vi "Repack Pixels_Pixel Bus to FIFO U1x8.vi"(10 "Input Valid":bool=TRUE, 11 "Pixel Bus In":T1={"Pixel Data"=[FALSE, FALSE, FALSE, FALSE, FALSE, FALSE, FALSE, FALSE], "DV"=[FALSE, FALSE, FALSE, FALSE, FALSE, FALSE, FALSE, FALSE], "EOL"=FALSE, "EOI"=FALSE, "Data Type"=enum."U1 x 8"}) -> (2 "Output Valid":bool, 3 "output array":bool[](array[boolean]))   [LabVIEW 2020, in "NI_VDM_FPGA_Basics.lvlib"]
uses:
  <vilib>/visionFPGA/NI_VDM_FPGA_Basics.lvlib
  <vilib>/visionFPGA/Controls/IMAQ FPGA Pixel Bus u1x8.ctl
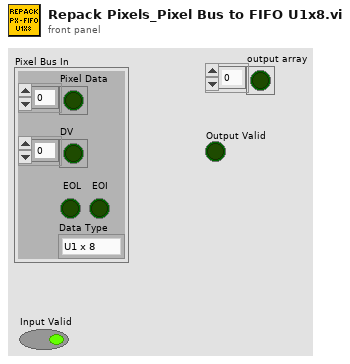
[diagram p1: front panel]
types:
  T1 = typedef "IMAQ FPGA Pixel Bus u1x8.ctl" = cluster{"Pixel Data":bool[], "DV":bool[], "EOL":bool, "EOI":bool, "Data Type":enum16{"U1 x 8"}}
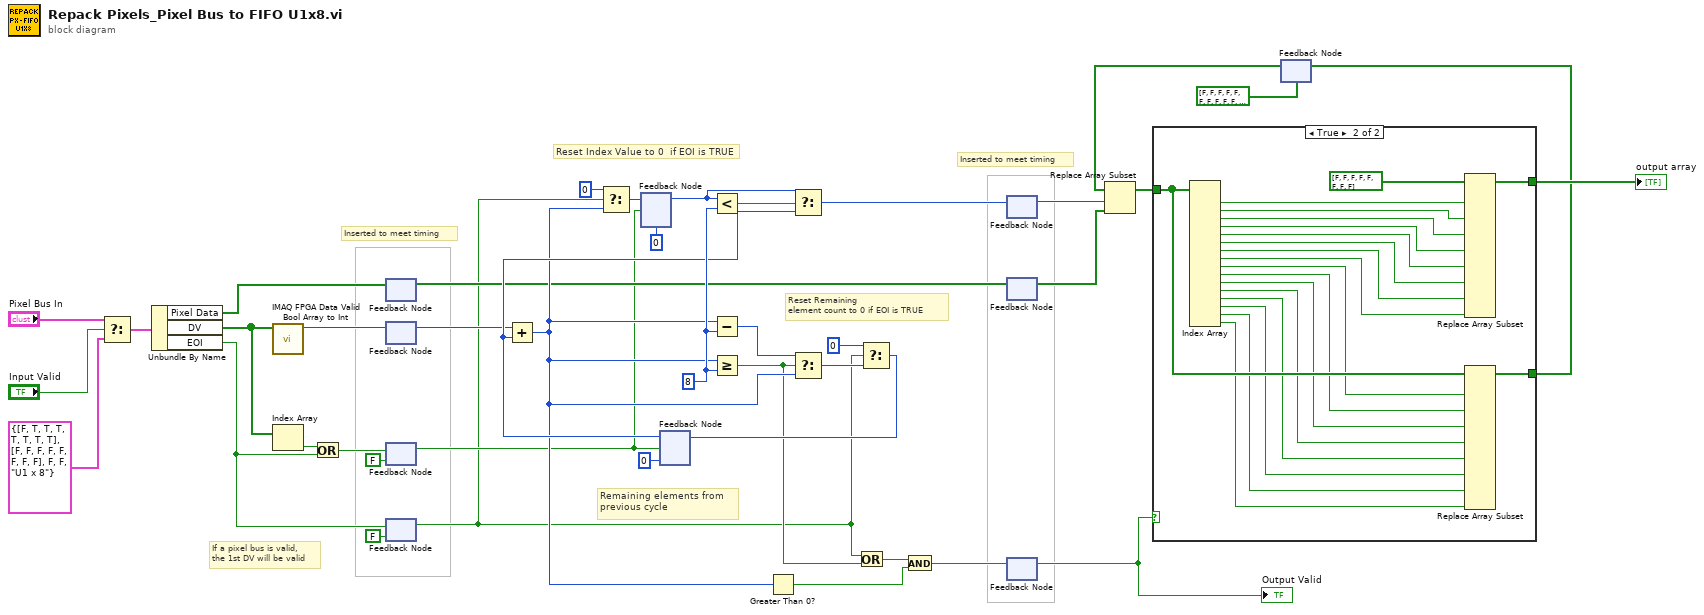
[diagram p0: block diagram]
diagram:
  w32 = u16 8 ("y")
  # "Inserted to meet timing"
  # "If a pixel bus is valid,\nthe 1st DV will be valid"
  # "Inserted to meet timing"
  # "Reset Remaining \nelement count to 0 if EOI is TRUE"
  # "Reset Index Value to 0  if EOI is TRUE"
  # "Remaining elements from \nprevious cycle"
  n1 = Select(t="Pixel Bus In", s="Input Valid", f=T1 {"Pixel Data"=[FALSE, TRUE, TRUE, TRUE, TRUE, TRUE, TRUE, TRUE], "DV"=[FALSE, FALSE, FALSE, FALSE, FALSE, FALSE, FALSE, FALSE], "EOL"=FALSE, "EOI"=FALSE, "Data Type"=enum."U1 x 8"} ("Pixel Bus In")) -> (s? t:f=w39:T1)
  n2 = Unbundle By Name(w39) -> ("Pixel Data"=w16:bool[], "DV"=w15:bool[], "EOI"=w9:bool)
  n3 = call <vilib>:"IMAQ FPGA Data Valid Bool Array to Int.vi"("DV In"=w15) -> ("Sum DV Out"=w28:u8)  [unwired: 10 in]
  n4 = Index Array(array=w15) -> (element=w17:bool)  [unwired: 1 in]
  n5 = Or(x=w17, y=w9) -> (x .or. y?=w12:bool)
  n6 = feedback-in #1(w16) -> ()
  n7 = feedback #1() -> (w14:bool[])  [unwired: 1 in]
  n8 = feedback-in #2(w28) -> ()
  n9 = feedback #2() -> (w13:u8)  [unwired: 1 in]
  n10 = feedback #3(FALSE) -> (w8:bool)
  n11 = feedback-in #3(w12) -> ()
  n12 = feedback #4(FALSE) -> (w1:bool)
  n13 = feedback-in #4(w9) -> ()
  n14 = feedback #5(u16 0 ("t")) -> (w31:u16)
  n15 = feedback #6(u16 0 ("t")) -> (w27:u16)
  n16 = Add(x=w13, y=w27) -> (x+y=w20:u16)
  n17 = Select(t=u16 0, s=w1, f=w20) -> (s? t:f=w22:u16)
  n18 = feedback-in #5(w22, w8) -> ()
  n19 = Less?(x=w31, y=w32) -> (x < y?=w29:bool)
  n20 = Subtract(x=w20, y=w32) -> (x-y=w33:u16)
  n21 = Greater Or Equal?(x=w20, y=w32) -> (x >= y?=w2:bool)
  n22 = Greater Than 0?(x=w20) -> (x > 0?=w19:bool)
  n23 = Select(t=w31, s=w29, f=w27) -> (s? t:f=w30:u16)
  n24 = Select(t=w33, s=w2, f=w20) -> (s? t:f=w25:u16)
  n25 = Or(x=w1, y=w2) -> (x .or. y?=w26:bool)
  n26 = Select(t=u16 0, s=w1, f=w25) -> (s? t:f=w23:u16)
  n27 = feedback-in #6(w23, w8) -> ()
  n28 = And(x=w26, y=w19) -> (x .and. y?=w42:bool)
  n29 = feedback-in #7(w30) -> ()
  n30 = feedback #7() -> (w6:u16)  [unwired: 1 in]
  n31 = feedback-in #8(w14) -> ()
  n32 = feedback #8() -> (w7:bool[])  [unwired: 1 in]
  n33 = feedback-in #9(w42) -> ()
  n34 = feedback #9() -> (w5:bool)  [unwired: 1 in]
  "Output Valid" <- w5
  n35 = feedback #10(bool[] [FALSE, FALSE, FALSE, FALSE, FALSE, FALSE, FALSE, FALSE, FALSE, FALSE, FALSE, FALSE, FALSE, FALSE, FALSE, FALSE] ("Pixel Data")) -> (w35:bool[])
  n36 = Replace Array Subset(array=w35, new element=w7, index=w6) -> (w34:bool[])
  n37 = case shown="True" w5 {
    tunnel: [w43 w63] -> w36
    tunnel: w34 -> [w43 w62]
    tunnel: [_ w45] -> w37
    frame False {
    }
    frame True {
      n38 = Index Array(array=w62) -> (element #1=w61:bool, element #2=w60:bool, element #3=w59:bool, element #4=w58:bool, element #5=w57:bool, element #6=w56:bool, element #7=w55:bool, element #8=w54:bool, element #9=w53:bool, element #10=w52:bool, element #11=w51:bool, element #12=w50:bool, element #13=w49:bool, element #14=w48:bool, element #15=w47:bool, element #16=w46:bool)  [unwired: 16 in]
      n39 = Replace Array Subset(array=bool[] [FALSE, FALSE, FALSE, FALSE, FALSE, FALSE, FALSE, FALSE] ("Pixel Data"), new element #1=w61, new element #2=w60, new element #3=w59, new element #4=w58, new element #5=w57, new element #6=w56, new element #7=w55, new element #8=w54) -> (w45:bool[])  [unwired: 8 in]
      n40 = Replace Array Subset(array=w62, new element #1=w53, new element #2=w52, new element #3=w51, new element #4=w50, new element #5=w49, new element #6=w48, new element #7=w47, new element #8=w46) -> (w63:bool[])  [unwired: 8 in]
    }
  }
  "output array" <- w37
  n41 = feedback-in #10(w36) -> ()
